vi "CameraControl.vi"(0 "Exposure Time":dbl=20011.0 min=61.0 max=16000000.0, 1 "Gain Selector":u32(ring)=1 items=["Sensor", "Digital"], 2 "Gain":dbl=1.0 min=1.0 max=4.0, 3 "Gain (Raw)":i64 min=0 max=384 step=1, 4 "Black Level Selector":u32(ring) items=["Analog"], 5 "Stop (F)":bool, 7 "error in":errorcluster, 8 "Black Level":dbl=240.0 min=0.0 max=511.0) -> (6 "Lost Packet Count":u32, 20 "Image Out":T1(plugin-control), 21 "All Image Buffers Out":T1[](array[typedef]), 26 "Stopped":bool, 27 "error out":errorcluster)   [LabVIEW 2016]
doc: "Creates, and edits acquisitions using the NI Vision Acquisition Express VI.\n\nThe NI Vision Acquisition Wizard is launched by placing the Express VI on the block diagram. Select an acquisition source and configure an acquisition using NI-IMAQ, NI-IMAQdx, or simulate an acquisition by reading an AVI or image files from a folder. After an acquisition is configured, select controls and indicators to be able to programmatically set in LabVIEW. Double-click the Vision Acquisition Express VI to edit the acquisition.\n\nNote: Any images created by the Express VI need to be disposed after use. Use the IMAQ Dispose.vi to cleanup the images output by the Express VI when they are no longer needed."
uses:
  <vilib>/vision/Image Controls.llb/IMAQ Image.ctl
  <vilib>/vision/driver/IMAQdx.llb/IMAQdx Buffer Number Mode.ctl
  <vilib>/vision/driver/NI_Vision_Acquisition_Software.lvlib
  <resource>/objmgr/imaqdx.rc
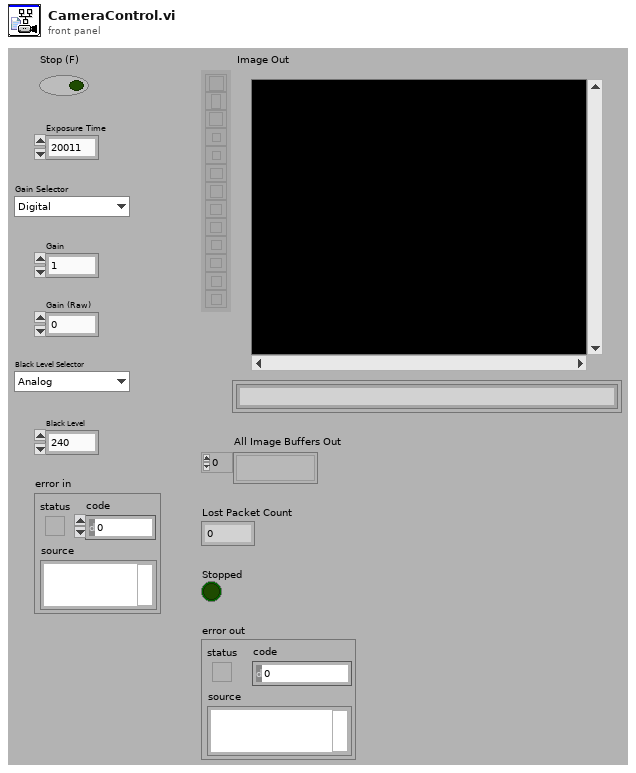
[diagram p1: front panel]
types:
  T1 = typedef "IMAQ Image.ctl" = refnum<image>
  T2 = typedef "NI_Vision_Acquisition_Software.lvlib/IMAQdx Buffer Number Mode.ctl" = enum32{"Next", "Last", "Buffer Number", "Every", "Last New"}
  T3 = typedef "IMAQdx.ctl" = refnum<k21>
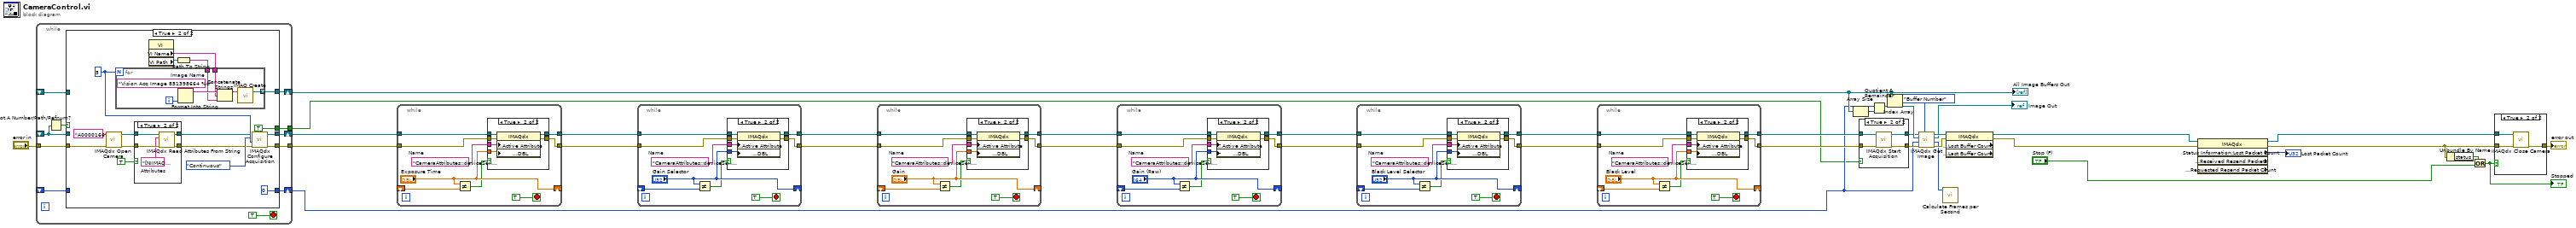
[diagram p0: block diagram]
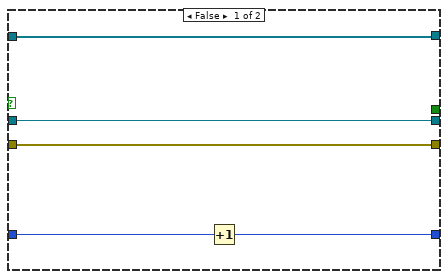
[diagram p10: hidden frame]
diagram:
  n1 = while {
    shift-right: [w48] -> w35
    shift-left: _ -> [w40]
    tunnel: [w47] -> w36
    tunnel: "error in" -> [w46]
    shift-right: [w44] -> w19
    shift-left: _ -> [w43]
    shift-right: [w42] -> w12
    shift-left: _ -> [w41]
    tunnel: [w38] -> w11
    stop <- TRUE stop-if-true
    n2 = Not A Number/Path/Refnum?(number/path/refnum=w40) -> (NaN/Path/Refnum?=w39:bool)
    n3 = case shown="True" w39 {
      tunnel: [w53 w68] -> w48
      tunnel: w40 -> [w53 _]
      tunnel: [w52 w67] -> w47
      tunnel: w46 -> [w52 w70]
      tunnel: [w51 w66] -> w44
      tunnel: w43 -> [w51 _]
      tunnel: [w49 0] -> w42
      tunnel: w41 -> [w50 _]
      tunnel: [_ TRUE] -> w38
      frame False {
        n4 = Increment(x=w50) -> (x+1=w49:i32)
      }
      frame True {
        w65 = u32 5 ("Number of Image Buffers")
        n5 = call <vilib>:"IMAQdx Open Camera.vi"("error in"=w70, "Session In"="A0000166" ("Interface Name")) -> ("error out"=w58:errorcluster, "Session Out"=w59:T3)  [unwired: 1 in, 7 out]
        n6 = case shown="True" TRUE ("Init Attributes") {
          tunnel: w59 -> [w72 w77]
          tunnel: w58 -> [w71 w76]
          tunnel: [w72 w74] -> w57
          tunnel: [w71 w73] -> w56
          frame False {
          }
          frame True {
            w75 = "[NIIMAQ_HEADER]\nType = 2\nVersion = 8\n\n[CAMERA_DATA]\nAcquisitionAttributes::AdvancedEthernet::BandwidthControl::DesiredPeakBandwidth = \"1000\"\nAcquisitionAttributes::AdvancedEthernet::Controller::DestinationMode = \"Unicast\"\nAcquisitionAttributes::AdvancedEthernet::Controller::DestinationMulticastAddress = \"239.192.0.1\"\nAcquisitionAttributes::AdvancedEthernet::EventParameters::EventsEnabled = \"true\"\nAcquisitionAttributes::AdvancedEthernet::EventParameters::MaxOutstandingEvents = \"50\"\nAcquisitionAttributes::AdvancedEthernet::FirewallTraversal::Enabled = \"true\"\nAcquisitionAttributes::AdvancedEthernet::FirewallTraversal::KeepAliveTime = \"30\"\nAcquisitionAttributes::AdvancedEthernet::ResendParameters::MaxResendsPerPacket = \"25\"\nAcquisitionAttributes::AdvancedEthernet::ResendParameters::MemoryWindowSize = \"1024\"\nAcquisitionAttributes::AdvancedEthernet::ResendParameters::MissingPacketTimeout = \"2\"\nAcquisitionAttributes::AdvancedEthernet::ResendParameters::NewPacketTimeout = \"100\"\nAcquisitionAttributes::AdvancedEthernet::ResendParameters::ResendBatchingPercentage = \"10\"\nAcquisitionAttributes::AdvancedEthernet::ResendParameters::ResendResponseTimeout = \"2\"\nAcquisitionAttributes::AdvancedEthernet::ResendParameters::ResendsEnabled = \"true\"\nAcquisitionAttributes::AdvancedEthernet::ResendParameters::ResendThresholdPercentage = \"5\"\nAcquisitionAttributes::AdvancedEthernet::ResendParameters::ResendTimerResolution = \"1\"\nAcquisitionAttributes::AdvancedEthernet::TestPacketParameters::MaxTestPacketRetries = \"1\"\nAcquisitionAttributes::AdvancedEthernet::TestPacketParameters::TestPacketEnabled = \"true\"\nAcquisitionAttributes::AdvancedEthernet::TestPacketParameters::TestPacketTimeout = \"250\"\nAcquisitionAttributes::AdvancedGenicam::CommandTimeout = \"100\"\nAcquisitionAttributes::Bayer::Algorithm = \"Bilinear\"\nAcquisitionAttributes::Bayer::GainB = \"1\"\nAcquisitionAttributes::Bayer::GainG = \"1\"\nAcquisitionAttributes::Bayer::GainR = \"1\"\nAcquisitionAttributes::Bayer::Pattern = \"Use hardware value\"\nAcquisitionAttributes::BitsPerPixel = \"Use hardware value\"\nAcquisitionAttributes::ChunkDataDecoding::ChunkDataDecodingEnabled = \"false\"\nAcquisitionAttributes::ChunkDataDecoding::MaximumChunkCopySize = \"64\"\nAcquisitionAttributes::IgnoreFirstFrame = \"false\"\nAcquisitionAttributes::ImageDecoderCopyMode = \"Auto\"\nAcquisitionAttributes::IncompleteBufferMode = \"Ignore\"\nAcquisitionAttributes::OutputImageType = \"Auto\"\nAcquisitionAttributes::OverwriteMode = \"Get Newest\"\nAcquisitionAttributes::PacketSize = \"8000\"\nAcquisitionAttributes::PixelSignedness = \"Use hardware value\"\nAcquisitionAttributes::ReceiveTimestampMode = \"None\"\nAcquisitionAttributes::ShiftPixelBits = \"false\"\nAcquisitionAttributes::SwapPixelBytes = \"false\"\nAcquisitionAttributes::Timeout = \"5000\"\nCameraAttributes::deviceCounterAndTimerControl::counterSelector = \"Counter 1\"\nCameraAttributes::deviceCounterAndTimerControl::counterMode = \"Off\"\nCameraAttributes::deviceCounterAndTimerControl::counterStartSource = \"Line 1\"\nCameraAttributes::deviceCounterAndTimerControl::counterStartLineActivation = \"Rising Edge\"\nCameraAttributes::deviceCounterAndTimerControl::counterIncrementalSource = \"Internal Clock\"\nCameraAttributes::deviceCounterAndTimerControl::counterResetSource = \"Reset Cmd\"\nCameraAttributes::deviceCounterAndTimerControl::counterDuration = \"1\"\nCameraAttributes::deviceCounterAndTimerControl::timerSelector = \"Timer 1\"\nCameraAttributes::deviceCounterAndTimerControl::timerMode = \"Off\"\nCameraAttributes::deviceCounterAndTimerControl::timerStartSource = \"Line 1\"\nCameraAttributes::deviceCounterAndTimerControl::timerStartLineActivation = \"Rising Edge\"\nCameraAttributes::deviceCounterAndTimerControl::timerDuration = \"1\"\nCameraAttributes::deviceSensorControl::AcquisitionFrameRate = \"24\"\nCameraAttributes::deviceSensorControl::BlackLevelSelector = \"Analog\"\nCameraAttributes::deviceSensorControl::BlackLevelRaw = \"240\"\nCameraAttributes::deviceSensorControl::exposureAlignment = \"Synchronous\"\nCameraAttributes::deviceSensorControl::ExposureMode = \"Timed\"\nCameraAttributes::deviceSensorControl::ExposureTime = \"20011\"\nCameraAttributes::deviceSensorControl::GainSelector = \"Sensor\"\nCameraAttributes::deviceSensorControl::Gain = \"1\"\nCameraAttributes::deviceSensorControl::GainSelector = \"Digital\"\nCameraAttributes::deviceSensorControl::Gain = \"1\"\nCameraAttributes::DigitalIOControl::LineSelector = \"Line 1\"\nCameraAttributes::DigitalIOControl::lineDetectionLevel = \"Threshold for TTL\"\nCameraAttributes::DigitalIOControl::LineInverter = \"false\"\nCameraAttributes::DigitalIOControl::lineDebouncingPeriod = \"0\"\nCameraAttributes::DigitalIOControl::LineSelector = \"Line 2\"\nCameraAttributes::DigitalIOControl::lineDetectionLevel = \"Threshold for TTL\"\nCameraAttributes::DigitalIOControl::LineInverter = \"false\"\nCameraAttributes::DigitalIOControl::lineDebouncingPeriod = \"0\"\nCameraAttributes::DigitalIOControl::LineSelector = \"Line 3\"\nCameraAttributes::DigitalIOControl::LineInverter = \"false\"\nCameraAttributes::DigitalIOControl::outputLineSource = \"Pulse On: Software Command\"\nCameraAttributes::DigitalIOControl::outputLinePulseDelay = \"0\"\nCameraAttributes::DigitalIOControl::outputLinePulseDuration = \"1\"\nCameraAttributes::DigitalIOControl::LineSelector = \"Line 4\"\nCameraAttributes::DigitalIOControl::LineInverter = \"false\"\nCameraAttributes::DigitalIOControl::outputLineSource = \"Pulse On: Software Command\"\nCameraAttributes::DigitalIOControl::outputLinePulseDelay = \"0\"\nCameraAttributes::DigitalIOControl::outputLinePulseDuration = \"1\"\nCameraAttributes::DigitalIOControl::LineSelector = \"Line 1\"\nCameraAttributes::DigitalIOControl::TriggerSelector = \"Single Frame Trigger(Start)\"\nCameraAttributes::DigitalIOControl::TriggerMode = \"Off\"\nCameraAttributes::DigitalIOControl::TriggerSelector = \"MultiFrame Trigger(Start)\"\nCameraAttributes::DigitalIOControl::TriggerMode = \"Off\"\nCameraAttributes::ImageFormatControl::Height = \"1080\"\nCameraAttributes::ImageFormatControl::OffsetX = \"0\"\nCameraAttributes::ImageFormatControl::OffsetY = \"0\"\nCameraAttributes::ImageFormatControl::PixelFormat = \"Monochrome 8-Bit\"\nCameraAttributes::ImageFormatControl::Width = \"1920\"\nCameraAttributes::TransportLayerControl::devicePacketResendBufferSize = \"24\"\n"  # Attributes
            n7 = call <vilib>:"IMAQdx Read Attributes From String.vi"("error in"=w76, "Attributes String In"=w75, "Session In"=w77) -> ("error out"=w73:errorcluster, "Session Out"=w74:T3)  [unwired: 7 out]
          }
        }
        n8 = property class="VI"() -> ("VI Name"=w61:string, "VI Path"=w62:path)  [unwired: 2 in, 2 out]
        n9 = Path To String(path=w62) -> (string=w60:string)
        n10 = for "For Loop_template0" {
          N: w65 -> [_]
          tunnel: [w84] -> w66 mode=indexing
          tunnel: w61 -> [w79]
          tunnel: w60 -> [w78]
          i -> [w83]
          w82 = "Vision Acq Image 851398664 %d"  # Image Name
          n11 = Format Into String(format string=w82, w83) -> (resulting string=w81:string)  [unwired: 2 in, 1 out]
          n12 = Concatenate Strings(w81, w79, w78) -> (w80:string)
          n13 = call "IMAQ Create"("Image Name"=w80) -> ("New Image"=w84:T1)  [unwired: 3 in, 2 out]
        }
        n14 = call <vilib>:"IMAQdx Configure Acquisition.vi"("error in"=w56, "Number of Buffers"=w65, "Continuous?"=enum32{"One Shot", "Continuous"}."Continuous" ("Mode"), "Session In"=w57) -> ("error out"=w67:errorcluster, "Session Out"=w68:T3)  [unwired: 6 out]
      }
    }
  }
  "All Image Buffers Out" <- w19
  n15 = while {
    tunnel: w36 -> [w93]
    tunnel: [w92] -> w33
    tunnel: w35 -> [w91]
    tunnel: [w90] -> w34
    shift-right: ["Exposure Time"] -> _
    shift-left: _ -> [w86]
    stop <- TRUE stop-if-true
    w89 = "CameraAttributes::deviceSensorControl::ExposureTime"  # Name
    n16 = Not Equal?(x="Exposure Time", y=w86) -> (x != y?=w85:bool)
    n17 = case shown="True" w85 {
      tunnel: w93 -> [w94 w101]
      tunnel: [w95 w100] -> w92
      tunnel: w91 -> [w95 w99]
      tunnel: [w94 w98] -> w90
      tunnel: w89 -> [_ w97]
      tunnel: "Exposure Time" -> [_ w96]
      frame False {
      }
      frame True {
        n18 = property class="IMAQdx"(reference=w99, error in=w101, "Camera Attributes:Active Attribute"=w97, "Camera Attributes:Value:DBL"=w96) -> (reference out=w100:T3, error out=w98:errorcluster)
      }
    }
  }
  n19 = while {
    tunnel: w34 -> [w110]
    tunnel: [w109] -> w31
    tunnel: w33 -> [w108]
    tunnel: [w107] -> w32
    shift-right: ["Gain Selector"] -> _
    shift-left: _ -> [w103]
    stop <- TRUE stop-if-true
    w106 = "CameraAttributes::deviceSensorControl::GainSelector"  # Name
    n20 = Not Equal?(x="Gain Selector", y=w103) -> (x != y?=w102:bool)
    n21 = case shown="True" w102 {
      tunnel: w110 -> [w111 w118]
      tunnel: [w112 w117] -> w109
      tunnel: w108 -> [w112 w116]
      tunnel: [w111 w115] -> w107
      tunnel: w106 -> [_ w114]
      tunnel: "Gain Selector" -> [_ w113]
      frame False {
      }
      frame True {
        n22 = property class="IMAQdx"(reference=w116, error in=w118, "Camera Attributes:Active Attribute"=w114, "Camera Attributes:Value:DBL"=w113) -> (reference out=w117:T3, error out=w115:errorcluster)
      }
    }
  }
  n23 = while {
    tunnel: w32 -> [w127]
    tunnel: [w126] -> w29
    tunnel: w31 -> [w125]
    tunnel: [w124] -> w30
    shift-right: ["Gain"] -> _
    shift-left: _ -> [w120]
    stop <- TRUE stop-if-true
    w123 = "CameraAttributes::deviceSensorControl::Gain"  # Name
    n24 = Not Equal?(x="Gain", y=w120) -> (x != y?=w119:bool)
    n25 = case shown="True" w119 {
      tunnel: w127 -> [w128 w135]
      tunnel: [w129 w134] -> w126
      tunnel: w125 -> [w129 w133]
      tunnel: [w128 w132] -> w124
      tunnel: w123 -> [_ w131]
      tunnel: "Gain" -> [_ w130]
      frame False {
      }
      frame True {
        n26 = property class="IMAQdx"(reference=w133, error in=w135, "Camera Attributes:Active Attribute"=w131, "Camera Attributes:Value:DBL"=w130) -> (reference out=w134:T3, error out=w132:errorcluster)
      }
    }
  }
  n27 = while {
    tunnel: w30 -> [w144]
    tunnel: [w143] -> w27
    tunnel: w29 -> [w142]
    tunnel: [w141] -> w28
    shift-right: ["Gain (Raw)"] -> _
    shift-left: _ -> [w137]
    stop <- TRUE stop-if-true
    w140 = "CameraAttributes::deviceSensorControl::GainRaw"  # Name
    n28 = Not Equal?(x="Gain (Raw)", y=w137) -> (x != y?=w136:bool)
    n29 = case shown="True" w136 {
      tunnel: w144 -> [w145 w152]
      tunnel: [w146 w151] -> w143
      tunnel: w142 -> [w146 w150]
      tunnel: [w145 w149] -> w141
      tunnel: w140 -> [_ w148]
      tunnel: "Gain (Raw)" -> [_ w147]
      frame False {
      }
      frame True {
        n30 = property class="IMAQdx"(reference=w150, error in=w152, "Camera Attributes:Active Attribute"=w148, "Camera Attributes:Value:DBL"=w147) -> (reference out=w151:T3, error out=w149:errorcluster)
      }
    }
  }
  n31 = while {
    tunnel: w28 -> [w161]
    tunnel: [w160] -> w25
    tunnel: w27 -> [w159]
    tunnel: [w158] -> w26
    shift-right: ["Black Level Selector"] -> _
    shift-left: _ -> [w154]
    stop <- TRUE stop-if-true
    w157 = "CameraAttributes::deviceSensorControl::BlackLevelSelector"  # Name
    n32 = Not Equal?(x="Black Level Selector", y=w154) -> (x != y?=w153:bool)
    n33 = case shown="True" w153 {
      tunnel: w161 -> [w162 w169]
      tunnel: [w163 w168] -> w160
      tunnel: w159 -> [w163 w167]
      tunnel: [w162 w166] -> w158
      tunnel: w157 -> [_ w165]
      tunnel: "Black Level Selector" -> [_ w164]
      frame False {
      }
      frame True {
        n34 = property class="IMAQdx"(reference=w167, error in=w169, "Camera Attributes:Active Attribute"=w165, "Camera Attributes:Value:DBL"=w164) -> (reference out=w168:T3, error out=w166:errorcluster)
      }
    }
  }
  n35 = while {
    tunnel: w26 -> [w178]
    tunnel: [w177] -> w15
    tunnel: w25 -> [w176]
    tunnel: [w175] -> w24
    shift-right: ["Black Level"] -> _
    shift-left: _ -> [w171]
    stop <- TRUE stop-if-true
    w174 = "CameraAttributes::deviceSensorControl::BlackLevel"  # Name
    n36 = Not Equal?(x="Black Level", y=w171) -> (x != y?=w170:bool)
    n37 = case shown="True" w170 {
      tunnel: w178 -> [w179 w186]
      tunnel: [w180 w185] -> w177
      tunnel: w176 -> [w180 w184]
      tunnel: [w179 w183] -> w175
      tunnel: w174 -> [_ w182]
      tunnel: "Black Level" -> [_ w181]
      frame False {
      }
      frame True {
        n38 = property class="IMAQdx"(reference=w184, error in=w186, "Camera Attributes:Active Attribute"=w182, "Camera Attributes:Value:DBL"=w181) -> (reference out=w185:T3, error out=w183:errorcluster)
      }
    }
  }
  n39 = Array Size(array=w19) -> (size(s)=w20:i32)
  n40 = case shown="True" w11 {
    tunnel: w15 -> [w188 w192]
    tunnel: w24 -> [w187 w191]
    tunnel: [w187 w190] -> w13
    tunnel: [w188 w189] -> w14
    frame False {
    }
    frame True {
      n41 = call <vilib>:"IMAQdx Start Acquisition.vi"("error in"=w191, "Session In"=w192) -> ("error out"=w190:errorcluster, "Session Out"=w189:T3)  [unwired: 8 out]
    }
  }
  n42 = Quotient & Remainder(x=w12, y=w20) -> (x-y*floor(x/y)=w18:i32)  [unwired: 1 out]
  n43 = Index Array(array=w19, index=w18) -> (element=w17:T1)
  n44 = call <vilib>:"IMAQdx Get Image.vi"("Buffer Number Mode (Next)"=IMAQdx_Buffer_Number_Mode."Buffer Number", "error in"=w13, "Buffer Number In"=w12, "Image In"=w17, "Session In"=w14) -> ("error out"=w22:errorcluster, "Buffer Number Out"=w10:u32, "Image Out"=→"Image Out":T1, "Session Out"=w23:T3)  [unwired: 3 out]
  n45 = call <vilib>:"Calculate Frames per Second.vi"("Buffer Number"=w10) -> ()  [unwired: 2 in, 9 out]
  n46 = property class="IMAQdx" props=["Status Information:Lost Buffer Count", "Status Information:Last Buffer Count"](reference=w23, error in=w22) -> (reference out=w8:T3, error out=w16:errorcluster)  [unwired: 2 out]
  n47 = property class="IMAQdx" props=["Status Information:Lost Packet Count", "Status Information:Received Resend Packets", "Status Information:Requested Resend Packet Count"](reference=w8, error in=w16) -> (reference out=w5:T3, error out=w7:errorcluster, "Status Information:Lost Packet Count"=→"Lost Packet Count":u32)  [unwired: 2 out]
  n48 = Unbundle By Name(w7) -> ("status"=w1:bool)
  n49 = Or(x=w1, y="Stop (F)") -> (x .or. y?=w2:bool)
  "Stopped" <- w2
  n50 = case "Case Structure_template1" shown="True" w2 {
    tunnel: [w193 w195] -> w4
    tunnel: w7 -> [w193 w196]
    tunnel: w5 -> [_ w194]
    frame False {
    }
    frame True {
      n51 = call <vilib>:"IMAQdx Close Camera.vi"("error in"=w196, "Session In"=w194) -> ("error out"=w195:errorcluster)  [unwired: 9 out]
    }
  }
  "error out" <- w4
